vi "cRIO - Parameter Druckregler.vi"(0 "Parameter Regler":sgl[][](array[numeric]), 2 "Istwerte Regler":sgl[][](array[numeric]), 9 "Aktion":T1) -> (10 "Istwerte Regler Kalter Block":sgl[][](array[numeric]), 11 "Istwerte Regler Gaskühler":sgl[][](array[numeric]), 12 "Aktive Regler":bool[](array[boolean]), 13 "Istwerte Regler Durchfluss":sgl[][](array[numeric]), 14 "Parameter Regler":sgl[][](array[numeric]), 15 "Istwerte Regler Druck PMA":sgl[][](array[numeric]), 16 "Istwerte Regler FT-IR":sgl[][](array[numeric]), 17 "Istwerte Regler Ausgang":sgl[][](array[numeric]), 18 "Istwerte Regler NDIR":sgl[][](array[numeric]), 19 "Istwerte Regler Filterblock":sgl[][](array[numeric]))   [LabVIEW 2020, in "Kommunikation mit cRIO.lvlib"]
uses:
  Kommunikation mit cRIO.lvlib
  Aktionen FGV Druckregler.ctl
  SysLog/SysLog Interface.ctl
  Seiten/Erweiterte Konfig/Erweiterte Konfig.lvlib
  Allgemein/allgemeine Sub-VIs.lvlib
  SysLog/SysLog.lvlib
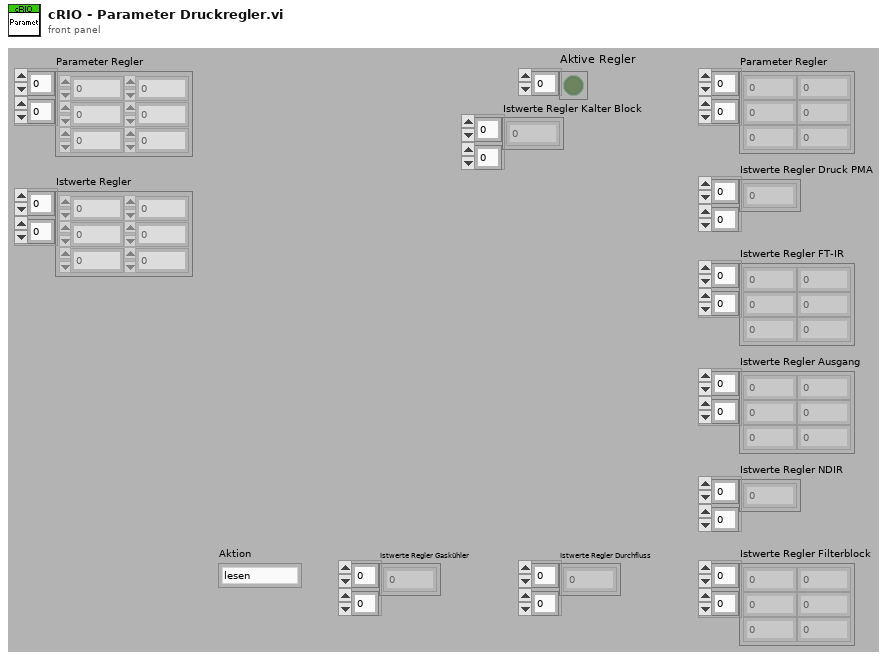
[diagram p1: front panel]
types:
  T1 = typedef "Kommunikation mit cRIO.lvlib/Aktionen FGV Druckregler.ctl" = enum16{"lesen", "Parameter", "Istwerte", "laden", "speichern"}
  T2 = typedef "SysLog.lvlib/SysLog Interface.ctl" = cluster{"FehlermeldungsCode":i32, "ErfolgsmeldungsCode":i32, "ParameterListenString":string, "Anzeige":bool, "SysLogIcon":enum16{"OK", "Warnung", "Fehler"}, "intern":bool}
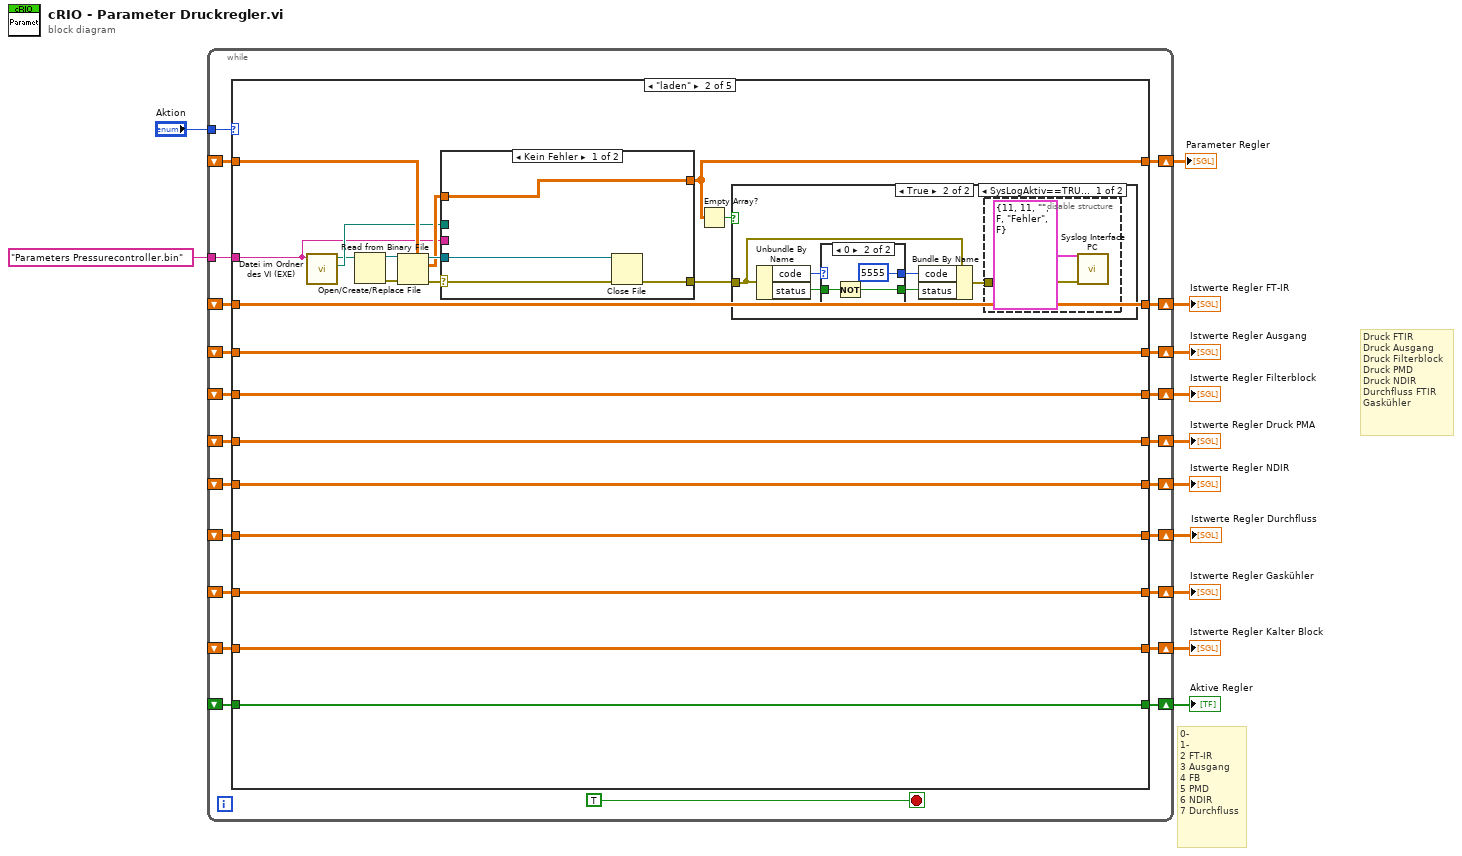
[diagram p0: block diagram]
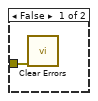
[diagram p3: hidden frame]
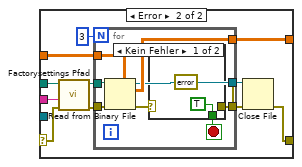
[diagram p6: hidden frame]
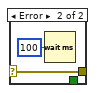
[diagram p7: hidden frame]
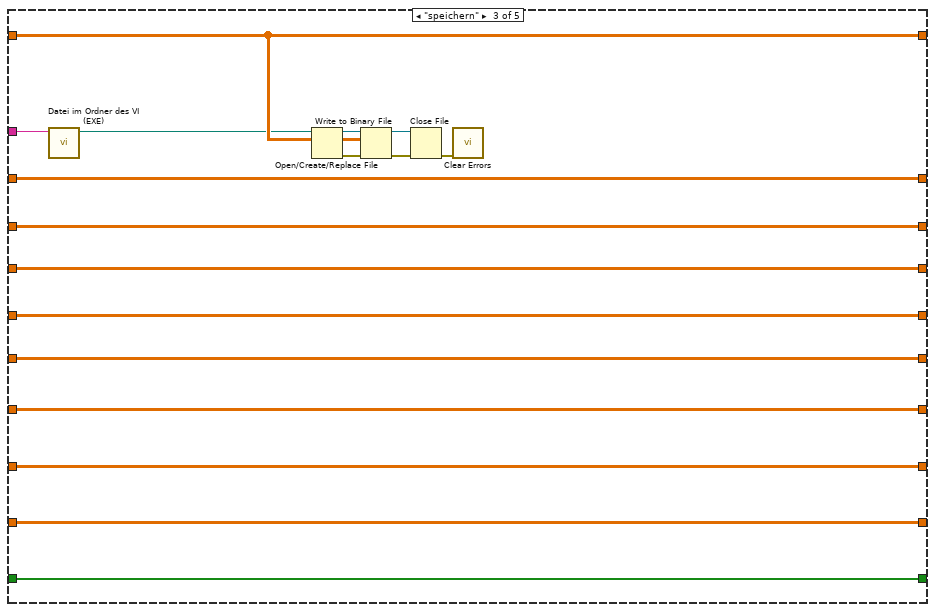
[diagram p8: hidden frame]
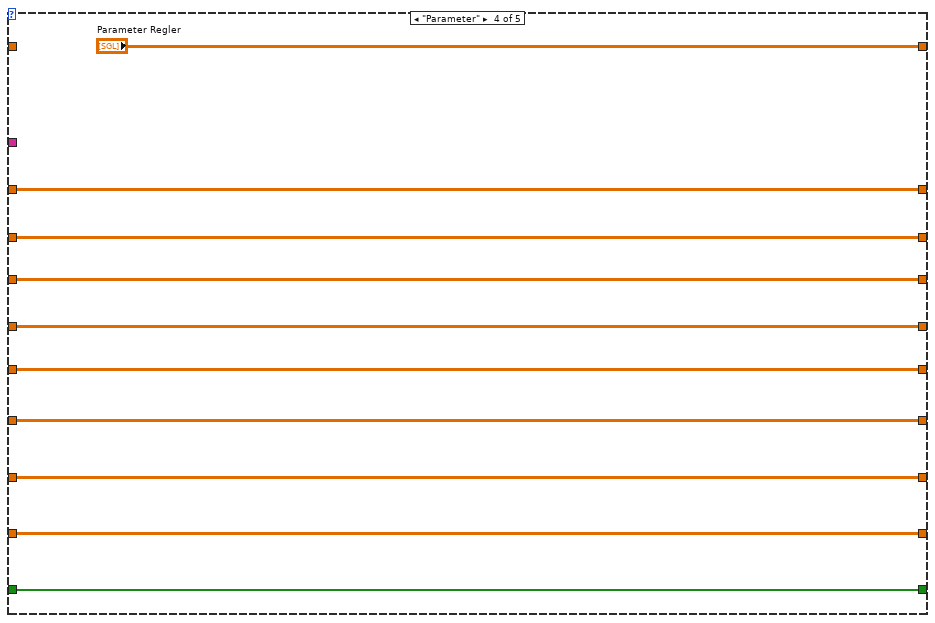
[diagram p9: hidden frame]
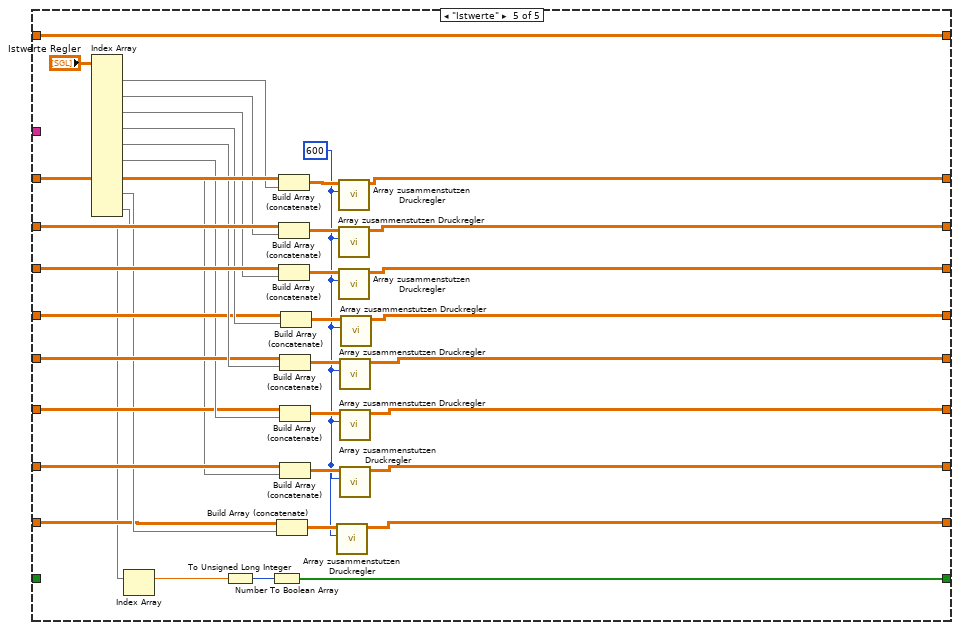
[diagram p10: hidden frame]
diagram:
  # "Druck FTIR\nDruck Ausgang\nDruck Filterblock\nDruck PMD\nDruck NDIR\nDurchfluss FTIR\nGaskühler"
  # "0-\n1-\n2 FT-IR\n3 Ausgang\n4 FB\n5 PMD\n6 NDIR\n7 Durchfluss"
  n1 = while {
    shift-right: [w34] -> w12
    shift-left: _ -> [w32]
    tunnel: "Aktion" -> [w33]
    shift-right: [w31] -> w10
    shift-left: _ -> [w30]
    shift-right: [w27] -> w9
    shift-left: _ -> [w28]
    shift-right: [w26] -> w8
    shift-left: _ -> [w29]
    shift-right: [w25] -> w7
    shift-left: _ -> [w24]
    shift-right: [w23] -> w6
    shift-left: _ -> [w22]
    shift-right: [w21] -> w5
    shift-left: _ -> [w20]
    shift-right: [w19] -> w4
    shift-left: _ -> [w18]
    shift-right: [w17] -> w3
    shift-left: _ -> [w16]
    shift-right: [w15] -> w2
    shift-left: _ -> [w14]
    tunnel: "Parameters Pressurecontroller.bin" ("Dateiname") -> [w13]
    stop <- TRUE stop-if-true
    n2 = case shown="\"laden\"" w33 {
      tunnel: [w45 w49 w114 "Parameter Regler" w173] -> w34
      tunnel: w32 -> [w45 w57 w114 _ w173]
      tunnel: [w44 w66 w124 w133 w168] -> w31
      tunnel: w30 -> [w44 w66 w124 w133 w172]
      tunnel: w29 -> [w42 w64 w122 w131 w165]
      tunnel: w28 -> [w43 w65 w123 w132 w164]
      tunnel: [w43 w65 w123 w132 w163] -> w27
      tunnel: [w42 w64 w122 w131 w162] -> w26
      tunnel: [w41 w63 w121 w130 w155] -> w25
      tunnel: w24 -> [w41 w63 w121 w130 w154]
      tunnel: [w40 w62 w120 w129 w153] -> w23
      tunnel: w22 -> [w40 w62 w120 w129 w152]
      tunnel: [w39 w61 w119 w128 w149] -> w21
      tunnel: w20 -> [w39 w61 w119 w128 w148]
      tunnel: [w38 w60 w118 w127 w146] -> w19
      tunnel: w18 -> [w38 w60 w118 w127 w145]
      tunnel: [w37 w59 w117 w126 w141] -> w17
      tunnel: w16 -> [w37 w59 w117 w126 _]
      tunnel: [w36 w58 w116 w125 w138] -> w15
      tunnel: w14 -> [w36 w58 w116 w125 w137]
      tunnel: w13 -> [_ w52 w115 _ _]
      frame "lesen", Default {
      }
      frame "laden" {
        n3 = call "Datei im Ordner des VI (EXE).vi"("Dateiname"=w52) -> ("Ordner des Haupt-VIs"=w53:path, "Dateipfad im Ordner des Haupt-VIs"=w48:path)  [unwired: 8 in, 1 out]
        n4 = Open/Create/Replace File(file path (use dialog)=w48) -> (refnum out=w47:refnum<file>, error out=w46:errorcluster)  [unwired: 5 in, 1 out]
        n5 = Read from Binary File(5:w57, 8:w46, 11:w47) -> (0:w56:errorcluster, 2:w54:sgl[][], 3:w55:refnum<file>)  [unwired: 4 out]
        n6 = case shown="Kein Fehler" w56 {
          selector: w56 -> [w83 w87]
          tunnel: w53 -> [_ w88]
          tunnel: w54 -> [w84 w86]
          tunnel: [w84 w94] -> w49
          tunnel: [w81 w92] -> w50
          tunnel: w55 -> [w82 _]
          tunnel: w52 -> [_ w85]
          frame No Error {
            n7 = Close File(refnum=w82, error in=w83) -> (error out=w81:errorcluster)  [unwired: 1 out]
          }
          frame Error {
            n8 = call "Factorysettings Pfad.vi"("error in (no error)"=w87, "Dateiname"=w85, "Ordner des Haupt-VIs"=w88) -> ("error out"=w89:errorcluster, "Pfad Factorysettings"=w90:path)  [unwired: 7 in]
            n9 = for {
              N: 3 -> [_]
              tunnel: w89 -> [w101]
              tunnel: w90 -> [w100]
              tunnel: [w99] -> w94
              tunnel: [w98] -> w93
              tunnel: [w97] -> w91
              tunnel: w86 -> [w96]
              stop <- w102 stop-if-true
              n10 = Read from Binary File(5:w96, 8:w101, 11:w100) -> (0:w103:errorcluster, 2:w99:sgl[][], 3:w97:refnum<file>)  [unwired: 3 in, 1 out]
              n11 = case shown="Kein Fehler" w103 {
                selector: w103 -> [_ w106]
                tunnel: [TRUE _] -> w102
                tunnel: [errorcluster {"status"=FALSE, "code"=0, "source"=""} ("error IO") w106] -> w98
                frame No Error {
                }
                frame Error {
                  n12 = Wait (ms)(milliseconds to wait=u32 100 ("Zu wartende ms")) -> ()  [unwired: 1 out]
                }
              }
            }
            n13 = Close File(refnum=w91, error in=w93) -> (error out=w92:errorcluster)  [unwired: 1 out]
          }
        }
        n14 = Empty Array?(array=w49) -> (empty?=w51:bool)
        n15 = case shown="True" w51 {
          tunnel: w50 -> [w67 w69]
          frame False {
            n16 = call <vilib>:"Clear Errors.vi"("error in (no error)"=w67) -> ()  [unwired: 5 in, 2 out]
          }
          frame True {
            n17 = Unbundle By Name(w69) -> ("code"=w73:i32, "status"=w72:bool)
            n18 = case shown="0" w73 {
              selector: w73 -> [w77 _]
              tunnel: [w77 5555 ("code")] -> w71
              tunnel: w72 -> [w76 w79]
              tunnel: [w76 w78] -> w70
              frame Default {
              }
              frame 0 {
                n19 = Not(x=w79) -> (.not. x?=w78:bool)
              }
            }
            n20 = Bundle By Name(cluster=w69, "code"=w71, "status"=w70) -> (w68:errorcluster)
            n21 = disable-structure shown="SysLogAktiv==TRUE" {
              disable-tunnel: w68 -> [w75 _]
              frame condition #0 (active) {
                n22 = call "Syslog Interface PC.vi"("Fehler (in)"=w75, "Cluster (in)"=T2 {"FehlermeldungsCode"=11, "ErfolgsmeldungsCode"=11, "ParameterListenString"="", "Anzeige"=FALSE, "SysLogIcon"=enum."Fehler", "intern"=FALSE}) -> ()  [unwired: 9 in, 1 out]
              }
              frame condition #1 {
              }
            }
          }
        }
      }
      frame "speichern" {
        n23 = call "Datei im Ordner des VI (EXE).vi"("Dateiname"=w115) -> ("Dateipfad im Ordner des Haupt-VIs"=w108:path)  [unwired: 8 in, 2 out]
        n24 = Open/Create/Replace File(file path (use dialog)=w108) -> (refnum out=w109:refnum<file>, error out=w110:errorcluster)  [unwired: 5 in, 1 out]
        n25 = Write to Binary File(file (use dialog)=w109, data=w114, error in=w110) -> (refnum out=w112:refnum<file>, error out=w113:errorcluster)  [unwired: 4 out]
        n26 = Close File(refnum=w112, error in=w113) -> (error out=w111:errorcluster)  [unwired: 1 out]
        n27 = call <vilib>:"Clear Errors.vi"("error in (no error)"=w111) -> ()  [unwired: 5 in, 2 out]
      }
      frame "Parameter" {
      }
      frame "Istwerte" {
        w135 = 600 ("Anzahl Elemente")
        n28 = Index Array(array="Istwerte Regler") -> (element #1=w170:sgl[], element #2=w161:sgl[], element #3=w160:sgl[], element #4=w157:sgl[], element #5=w156:sgl[], element #6=w150:sgl[], element #7=w144:sgl[], element #8=w139:sgl[], element #9=w136:sgl[])  [unwired: 18 in]
        n29 = Index Array(array=w136) -> (element=w142:sgl)  [unwired: 1 in]
        n30 = To Unsigned Long Integer(number=w142) -> (unsigned 32bit integer=w143:u32)
        n31 = Number To Boolean Array(number=w143) -> (Boolean array=w141:bool[])
        n32 = Build Array (concatenate)(w137, w139) -> (w140:sgl[][])
        n33 = Build Array (concatenate)(w172, w170) -> (w169:sgl[][])
        n34 = Build Array (concatenate)(w164, w161) -> (w167:sgl[][])
        n35 = Build Array (concatenate)(w165, w160) -> (w166:sgl[][])
        n36 = Build Array (concatenate)(w152, w156) -> (w158:sgl[][])
        n37 = Build Array (concatenate)(w148, w150) -> (w151:sgl[][])
        n38 = Build Array (concatenate)(w145, w144) -> (w147:sgl[][])
        n39 = Build Array (concatenate)(w154, w157) -> (w159:sgl[][])
        n40 = call "Array zusammenstutzen Druckregler.vi"("Anzahl Elemente"=w135, "Daten 1"=w140) -> ("Daten 1"=w138:sgl[][])  [unwired: 9 in]
        n41 = call "Array zusammenstutzen Druckregler.vi"("Anzahl Elemente"=w135, "Daten 1"=w169) -> ("Daten 1"=w168:sgl[][])  [unwired: 9 in]
        n42 = call "Array zusammenstutzen Druckregler.vi"("Anzahl Elemente"=w135, "Daten 1"=w167) -> ("Daten 1"=w163:sgl[][])  [unwired: 9 in]
        n43 = call "Array zusammenstutzen Druckregler.vi"("Anzahl Elemente"=w135, "Daten 1"=w166) -> ("Daten 1"=w162:sgl[][])  [unwired: 9 in]
        n44 = call "Array zusammenstutzen Druckregler.vi"("Anzahl Elemente"=w135, "Daten 1"=w158) -> ("Daten 1"=w153:sgl[][])  [unwired: 9 in]
        n45 = call "Array zusammenstutzen Druckregler.vi"("Anzahl Elemente"=w135, "Daten 1"=w151) -> ("Daten 1"=w149:sgl[][])  [unwired: 9 in]
        n46 = call "Array zusammenstutzen Druckregler.vi"("Anzahl Elemente"=w135, "Daten 1"=w147) -> ("Daten 1"=w146:sgl[][])  [unwired: 9 in]
        n47 = call "Array zusammenstutzen Druckregler.vi"("Anzahl Elemente"=w135, "Daten 1"=w159) -> ("Daten 1"=w155:sgl[][])  [unwired: 9 in]
      }
    }
  }
  "Parameter Regler" <- w12
  "Istwerte Regler FT-IR" <- w10
  "Istwerte Regler Filterblock" <- w8
  "Istwerte Regler Ausgang" <- w9
  "Istwerte Regler Druck PMA" <- w7
  "Istwerte Regler NDIR" <- w6
  "Istwerte Regler Durchfluss" <- w5
  "Istwerte Regler Gaskühler" <- w4
  "Aktive Regler" <- w3
  "Istwerte Regler Kalter Block" <- w2
